vi "MischerMonitor.vi"() -> ()   [LabVIEW 2018]
uses:
  Utility/Monitor Communication/Mischer/Mischer-Cluster.ctl
  Global/Global Variables/Data_Display_global.vi
panel:
  out "Mischer Monitor":T1
  # "2"
  # "to Condenser"
  # "1"
  # "7"
  # "From Still"
  # "5"
  # "Mischer\nEinheit"
  # "12"
  # "Cold\nTrap"
  # "Dump"
  # "9"
  # "8"
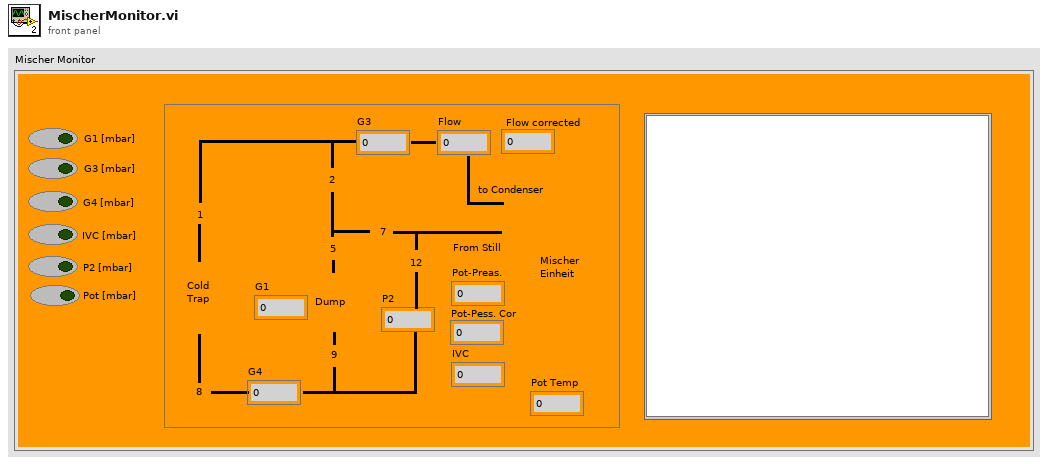
[diagram p1: front panel]
types:
  T1 = typedef "Mischer-Cluster.ctl" = cluster{"G4":dbl, "G1":dbl, "P2":dbl, "G3":dbl, "Flow":dbl, "Pot-Preas.":dbl, "IVC":dbl, "G1 [mbar]":bool, "G3 [mbar]":bool, "G4 [mbar]":bool, "IVC [mbar]":bool, "P2 [mbar] ":bool, "Flow corrected":dbl, "Pot-Pess. Cor":dbl, "Pot Temp":dbl, "Pot [mbar]":bool, "Plot":dbl[][]}
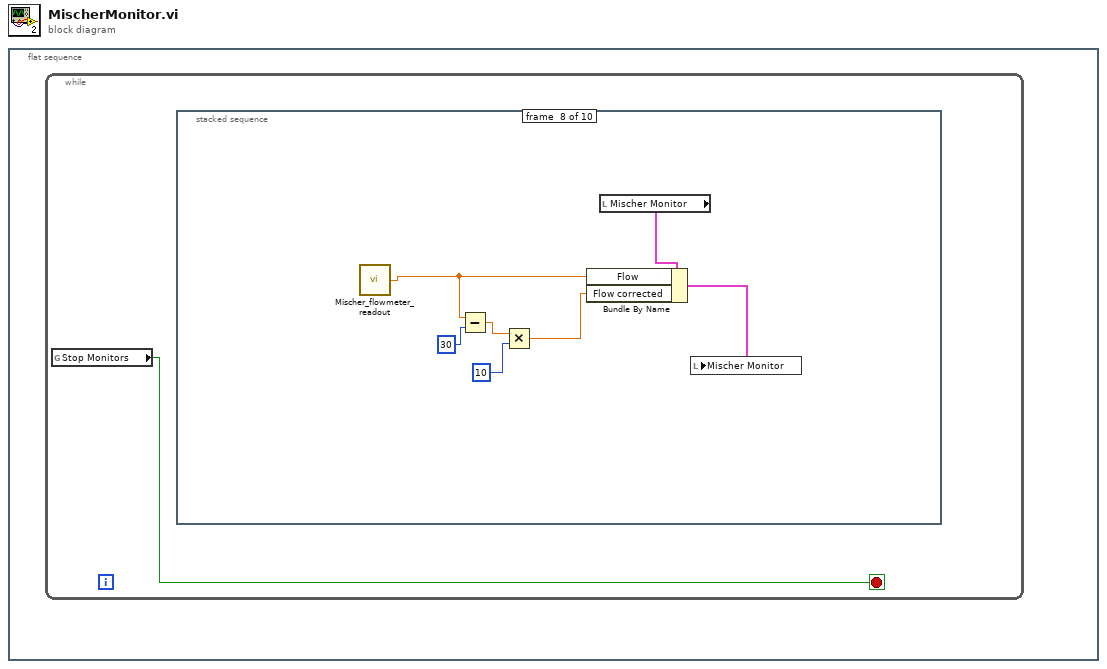
[diagram p0: block diagram]
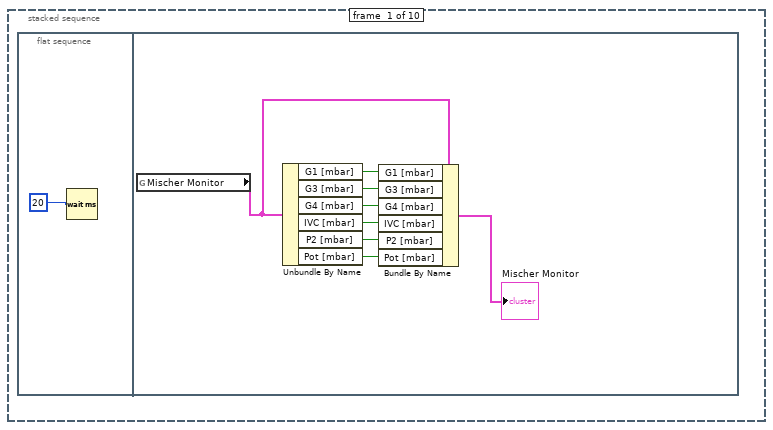
[diagram p2: hidden frame]
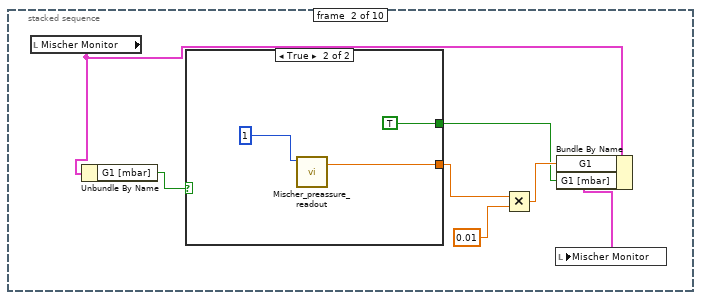
[diagram p3: hidden frame]
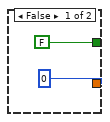
[diagram p4: hidden frame]
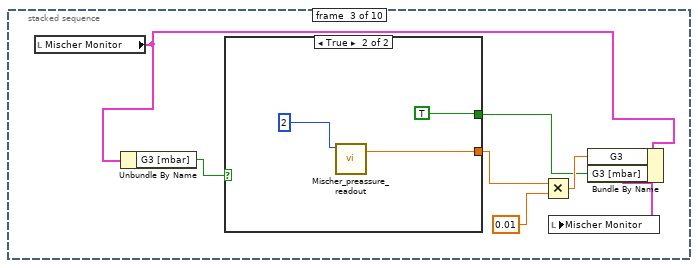
[diagram p5: hidden frame]
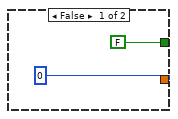
[diagram p6: hidden frame]
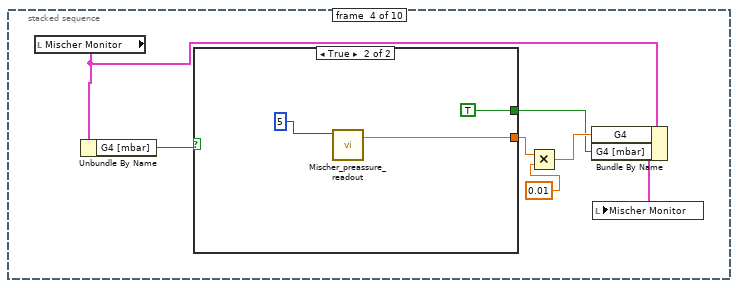
[diagram p7: hidden frame]
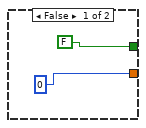
[diagram p8: hidden frame]
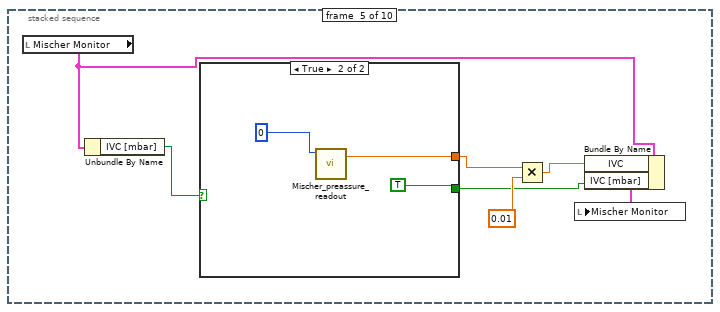
[diagram p9: hidden frame]
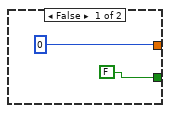
[diagram p10: hidden frame]
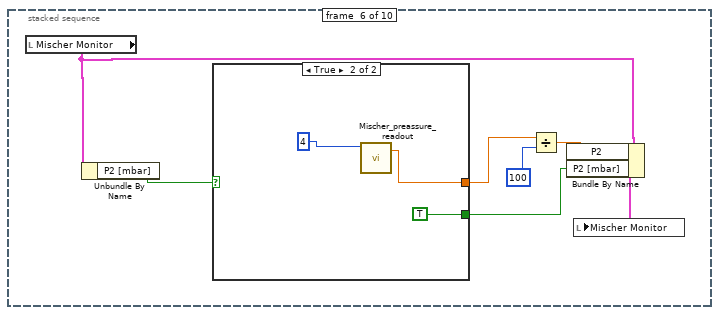
[diagram p11: hidden frame]
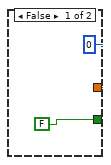
[diagram p12: hidden frame]
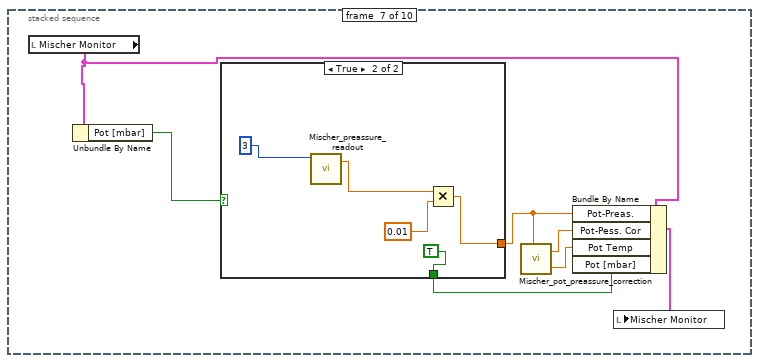
[diagram p13: hidden frame]
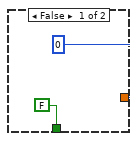
[diagram p14: hidden frame]
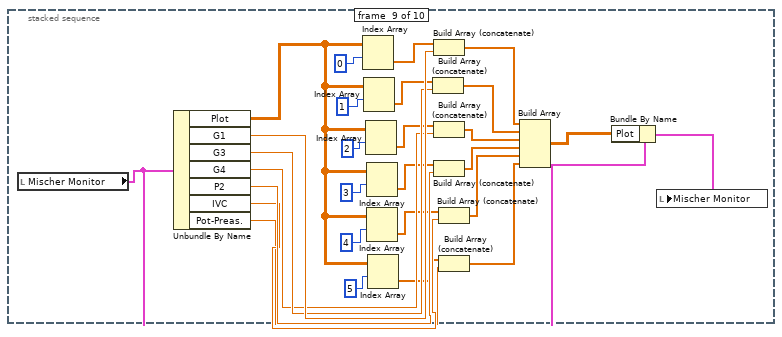
[diagram p15: hidden frame]
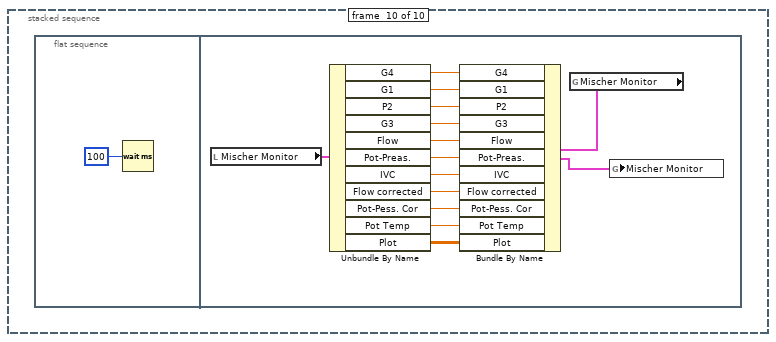
[diagram p16: hidden frame]
diagram:
  n1 = flat-sequence {
    frame #0 {
      n2 = while {
        stop <- w1 stop-if-true
        n3 = global read "Data_Display_global.vi" "Stop Monitors"() -> (w1:bool)
        n4 = stacked-sequence {
          frame #0 {
            n5 = flat-sequence {
              frame #0 {
                n6 = Wait (ms)(milliseconds to wait=20) -> ()  [unwired: 1 out]
              }
              frame #1 {
                n7 = global read "Data_Display_global.vi" "Mischer Monitor"() -> (w3:T1)
                n8 = Unbundle By Name(w3) -> ("G1 [mbar]"=w9:bool, "G3 [mbar]"=w8:bool, "G4 [mbar]"=w7:bool, "IVC [mbar]"=w6:bool, "P2 [mbar]"=w5:bool, "Pot [mbar]"=w4:bool)
                n9 = Bundle By Name(cluster=w3, "G1 [mbar]"=w9, "G3 [mbar]"=w8, "G4 [mbar]"=w7, "IVC [mbar]"=w6, "P2 [mbar]"=w5, "Pot [mbar]"=w4) -> (→"Mischer Monitor":T1)
              }
            }
          }
          frame #1 {
            n10 = local read "Mischer Monitor"() -> (w11:T1)
            n11 = Unbundle By Name(w11) -> ("G1 [mbar]"=w17:bool)
            n12 = case shown="True" w17 {
              tunnel: [0 w21] -> w15
              tunnel: [FALSE TRUE] -> w12
              frame False {
              }
              frame True {
                n13 = call "Mischer_preassure_readout.vi"("Gauge Number (1)"=1) -> ("Reading [V/mbar]"=w21:dbl)  [unwired: 6 in]
              }
            }
            n14 = Multiply(x=w15, y=0.01) -> (x*y=w13:dbl)
            n15 = Bundle By Name(cluster=w11, "G1"=w13, "G1 [mbar]"=w12) -> (w16:T1)
            n16 = local write "Mischer Monitor"(w16) -> ()
          }
          frame #2 {
            n17 = local read "Mischer Monitor"() -> (w23:T1)
            n18 = Unbundle By Name(w23) -> ("G3 [mbar]"=w29:bool)
            n19 = case shown="True" w29 {
              tunnel: [0 w33] -> w27
              tunnel: [FALSE TRUE] -> w24
              frame False {
              }
              frame True {
                n20 = call "Mischer_preassure_readout.vi"("Gauge Number (1)"=2) -> ("Reading [V/mbar]"=w33:dbl)  [unwired: 6 in]
              }
            }
            n21 = Multiply(x=w27, y=0.01) -> (x*y=w25:dbl)
            n22 = Bundle By Name(cluster=w23, "G3"=w25, "G3 [mbar]"=w24) -> (w28:T1)
            n23 = local write "Mischer Monitor"(w28) -> ()
          }
          frame #3 {
            n24 = local read "Mischer Monitor"() -> (w35:T1)
            n25 = Unbundle By Name(w35) -> ("G4 [mbar]"=w41:bool)
            n26 = case shown="True" w41 {
              tunnel: [0 w45] -> w39
              tunnel: [FALSE TRUE] -> w36
              frame False {
              }
              frame True {
                n27 = call "Mischer_preassure_readout.vi"("Gauge Number (1)"=5) -> ("Reading [V/mbar]"=w45:dbl)  [unwired: 6 in]
              }
            }
            n28 = Multiply(x=w39, y=0.01) -> (x*y=w37:dbl)
            n29 = Bundle By Name(cluster=w35, "G4"=w37, "G4 [mbar]"=w36) -> (w40:T1)
            n30 = local write "Mischer Monitor"(w40) -> ()
          }
          frame #4 {
            n31 = local read "Mischer Monitor"() -> (w47:T1)
            n32 = Unbundle By Name(w47) -> ("IVC [mbar]"=w53:bool)
            n33 = case shown="True" w53 {
              tunnel: [0 w57] -> w52
              tunnel: [FALSE TRUE] -> w48
              frame False {
              }
              frame True {
                n34 = call "Mischer_preassure_readout.vi"("Gauge Number (1)"=0) -> ("Reading [V/mbar]"=w57:dbl)  [unwired: 6 in]
              }
            }
            n35 = Multiply(x=w52, y=0.01) -> (x*y=w49:dbl)
            n36 = Bundle By Name(cluster=w47, "IVC"=w49, "IVC [mbar]"=w48) -> (w50:T1)
            n37 = local write "Mischer Monitor"(w50) -> ()
          }
          frame #5 {
            n38 = local read "Mischer Monitor"() -> (w59:T1)
            n39 = Unbundle By Name(w59) -> ("P2 [mbar]"=w65:bool)
            n40 = case shown="True" w65 {
              tunnel: [0 w69] -> w64
              tunnel: [FALSE TRUE] -> w60
              frame False {
              }
              frame True {
                n41 = call "Mischer_preassure_readout.vi"("Gauge Number (1)"=4) -> ("Reading [V/mbar]"=w69:dbl)  [unwired: 6 in]
              }
            }
            n42 = Divide(x=w64, y=100) -> (x/y=w61:dbl)
            n43 = Bundle By Name(cluster=w59, "P2"=w61, "P2 [mbar]"=w60) -> (w62:T1)
            n44 = local write "Mischer Monitor"(w62) -> ()
          }
          frame #6 {
            n45 = local read "Mischer Monitor"() -> (w71:T1)
            n46 = Unbundle By Name(w71) -> ("Pot [mbar]"=w77:bool)
            n47 = case shown="True" w77 {
              tunnel: [0 w81] -> w75
              tunnel: [FALSE TRUE] -> w72
              frame False {
              }
              frame True {
                n48 = call "Mischer_preassure_readout.vi"("Gauge Number (1)"=3) -> ("Reading [V/mbar]"=w83:dbl)  [unwired: 6 in]
                n49 = Multiply(x=w83, y=0.01) -> (x*y=w81:dbl)
              }
            }
            n50 = call "Mischer_pot_preassure_correction.vi"("Pot [mbar]"=w75) -> ("Pot corrected [mbar]"=w74:dbl, "TemperaturePot [K]"=w73:dbl)
            n51 = Bundle By Name(cluster=w71, "Pot-Preas."=w75, "Pot-Pess. Cor"=w74, "Pot Temp"=w73, "Pot [mbar]"=w72) -> (w76:T1)
            n52 = local write "Mischer Monitor"(w76) -> ()
          }
          frame #7 {
            n53 = call "Mischer_flowmeter_readout.vi"() -> ("Flow \n[µmol/sec He-3*(100]"=w88:dbl)  [unwired: 6 in]
            n54 = Subtract(x=w88, y=30) -> (x-y=w86:dbl)
            n55 = Multiply(x=w86, y=10) -> (x*y=w85:dbl)
            n56 = local read "Mischer Monitor"() -> (w91:T1)
            n57 = Bundle By Name(cluster=w91, "Flow"=w88, "Flow corrected"=w85) -> (w90:T1)
            n58 = local write "Mischer Monitor"(w90) -> ()
          }
          frame #8 {
            n59 = local read "Mischer Monitor"() -> (w94:T1)
            n60 = Unbundle By Name(w94) -> ("Plot"=w119:dbl[][], "G1"=w112:dbl, "G3"=w111:dbl, "G4"=w110:dbl, "P2"=w109:dbl, "IVC"=w108:dbl, "Pot-Preas."=w107:dbl)
            n61 = Index Array(array=w119, index (row)=0) -> (element=w106:dbl[])  [unwired: 1 in]
            n62 = Index Array(array=w119, index (row)=1) -> (element=w105:dbl[])  [unwired: 1 in]
            n63 = Index Array(array=w119, index (row)=2) -> (element=w104:dbl[])  [unwired: 1 in]
            n64 = Index Array(array=w119, index (row)=3) -> (element=w103:dbl[])  [unwired: 1 in]
            n65 = Index Array(array=w119, index (row)=4) -> (element=w102:dbl[])  [unwired: 1 in]
            n66 = Index Array(array=w119, index (row)=5) -> (element=w101:dbl[])  [unwired: 1 in]
            n67 = Build Array (concatenate)(w105, w111) -> (w99:dbl[])
            n68 = Build Array (concatenate)(w106, w112) -> (w100:dbl[])
            n69 = Build Array (concatenate)(w104, w110) -> (w98:dbl[])
            n70 = Build Array (concatenate)(w103, w109) -> (w97:dbl[])
            n71 = Build Array (concatenate)(w102, w108) -> (w96:dbl[])
            n72 = Build Array (concatenate)(w101, w107) -> (w95:dbl[])
            n73 = Build Array(w100, w99, w98, w97, w96, w95) -> (w92:dbl[][])
            n74 = Bundle By Name(cluster=w94, "Plot"=w92) -> (w93:T1)
            n75 = local write "Mischer Monitor"(w93) -> ()
          }
          frame #9 {
            n76 = flat-sequence {
              frame #0 {
                n77 = Wait (ms)(milliseconds to wait=100) -> ()  [unwired: 1 out]
              }
              frame #1 {
                n78 = local read "Mischer Monitor"() -> (w134:T1)
                n79 = Unbundle By Name(w134) -> ("G4"=w131:dbl, "G1"=w130:dbl, "P2"=w129:dbl, "G3"=w128:dbl, "Flow"=w127:dbl, "Pot-Preas."=w126:dbl, "IVC"=w125:dbl, "Flow corrected"=w124:dbl, "Pot-Pess. Cor"=w123:dbl, "Pot Temp"=w122:dbl, "Plot"=w121:dbl[][])
                n80 = global read "Data_Display_global.vi" "Mischer Monitor"() -> (w132:T1)
                n81 = Bundle By Name(cluster=w132, "G4"=w131, "G1"=w130, "P2"=w129, "G3"=w128, "Flow"=w127, "Pot-Preas."=w126, "IVC"=w125, "Flow corrected"=w124, "Pot-Pess. Cor"=w123, "Pot Temp"=w122, "Plot"=w121) -> (w133:T1)
                n82 = global write "Data_Display_global.vi" "Mischer Monitor"(w133) -> ()
              }
            }
          }
        }
      }
    }
  }
